vi "RT - Pumps State Change.vi"(8 "error in":errorcluster, 9 "Pumps State":bool[](array[boolean]), 10 "Pumps State In":bool[](array[boolean])=[FALSE, FALSE, FALSE, FALSE, FALSE], 11 "Queue in":refnum<queue>) -> (0 "error out":errorcluster, 2 "Pumps State Out":bool[](array[boolean]))   [LabVIEW 2018]
uses:
  Message Queue/Message Cluster.ctl
  Message Queue/Message.ctl
  Controls/Pumps State Change.ctl
  Message Queue/Message Queue.lvlib
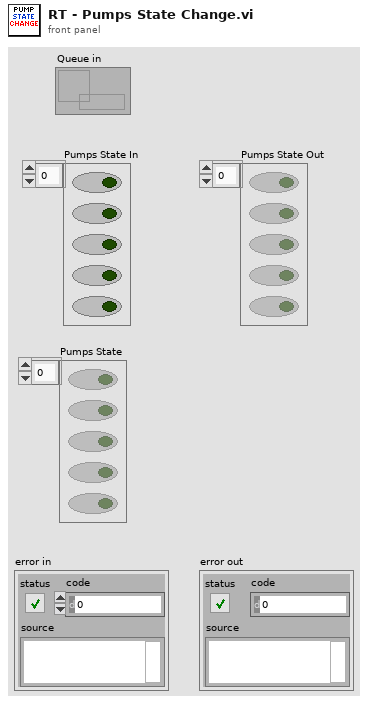
[diagram p1: front panel]
types:
  T1 = typedef "Message Queue.lvlib/Message.ctl" = enum16{"Initialize", "Initialize UI Refs", "Disable Controls", "Enable UI Controls", "Connect RT", "Get Control Mode from RT", "Send Control Mode to UI", "Update Control Mode", "Get Config from RT", "Send Config to UI", "Update Parameters", "Change Parameters", "Calibrate Config", "Update Calibration", "Change Valve State", "Get Valve Status from RT", "Send Valve Status to UI", "Update Valve Status", "Inital UI Values", "Disconnect RT", "Close Connection", "Disconnect UI", "Run Mode", "Stop ALL", "Change Control Mode", "Skid Manual", "Computer Manual", "Step Automated", "Fully Automated", "Reset", "Pumps Command", "Pump State Changed", "Critical Error", "Log-Only Error", "Non-Critical Error", "RT Error", "Update System Status", "Update DI Status", "Clear System Status", "Update Warning", "Clear Warning", "Upate Timeout", "Update Reset Status", "Waiting", "Verify Password", "Manual Cleaning Process", "Update Manual Cleaning Process", "Cal - Body", "Cal - US", "Cal - Update Parameters", "AddSub - BleedValve", "AddSub - TCValve", "AddSub - ABValve", "AddSub - TriplexPump", "Propotional Update", "Exit", "---Copy This Frame---"}
  T2 = typedef "Pumps State Change.ctl" = cluster{"Pump":enum16{"Pump 1", "Pump 2", "Pump 3", "Pump 4", "Pump 5"}, "On/Off":bool}
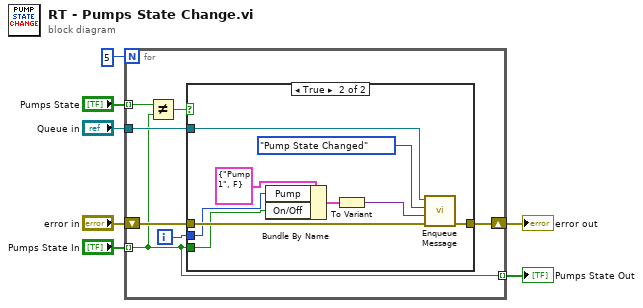
[diagram p0: block diagram]
diagram:
  n1 = for {
    N: 5 -> [_]
    tunnel: "Pumps State" -> [w14] mode=indexing
    tunnel: "Pumps State In" -> [w8] mode=indexing
    tunnel: "Queue in" -> [w12]
    shift-right: [w9] -> w6
    shift-left: "error in" -> [w10]
    tunnel: [w8] -> w7 mode=indexing
    i -> [w11]
    n2 = Not Equal?(x=w14, y=w8) -> (x != y?=w13:bool)
    n3 = case shown="True" w13 {
      tunnel: w8 -> [_ w19]
      tunnel: w12 -> [_ w24]
      tunnel: w11 -> [_ w17]
      tunnel: w10 -> [w15 w23]
      tunnel: [w15 w22] -> w9
      frame False {
      }
      frame True {
        n4 = Bundle By Name(cluster=T2 {"Pump"=enum."Pump 1", "On/Off"=FALSE} ("Pump State Change"), "Pump"=w17, "On/Off"=w19) -> (w18:T2)
        n5 = To Variant(anything=w18) -> (Variant=w21:variant)
        n6 = call "Enqueue Message.vi"("error in (no error)"=w23, "Message Data"=w21, "Message"=Message."Pump State Changed", "Message Queue"=w24) -> ("error out"=w22:errorcluster)  [unwired: 6 in, 1 out]
      }
    }
  }
  "Pumps State Out" <- w7
  "error out" <- w6
